vi "Video Settings.vi"(11 "Codec Names":string[](array[string])) -> (0 "Image Width":i32, 1 "Image Height":i32, 2 "Codec Name":string, 3 "AVI fps":u32=5)   [LabVIEW 2013]
panel:
  in  "Image Width":i32
  in  "Image Height":i32
  in  "AVI fps":u32=5
  in  "Codec Index":i32=1
  in  "stop":bool
  # "Enter Video Settings and\nthen Accept."
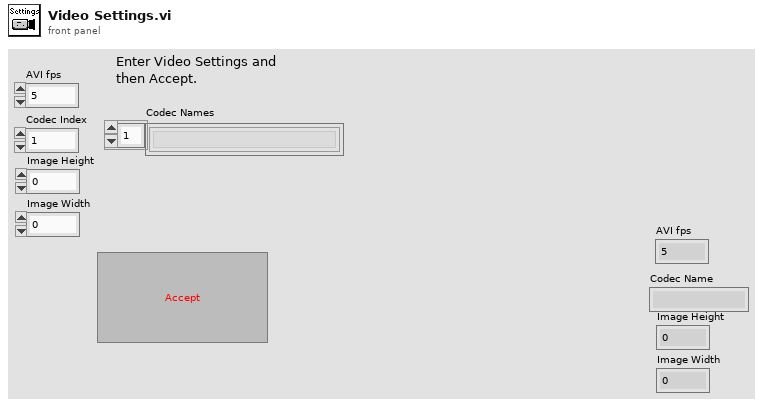
[diagram p1: front panel]
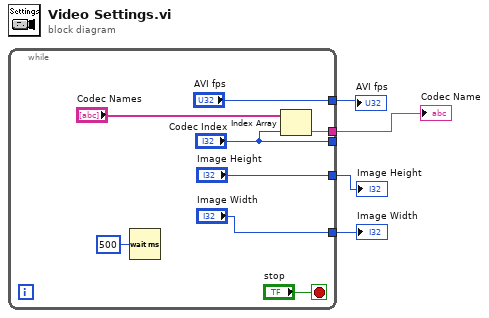
[diagram p0: block diagram]
diagram:
  n1 = while {
    tunnel: ["AVI fps"] -> w4
    tunnel: ["Codec Index"] -> _
    tunnel: ["Image Height"] -> w3
    tunnel: ["Image Width"] -> w2
    tunnel: [w5] -> w1
    stop <- "stop" stop-if-true
    n2 = Wait (ms)(milliseconds to wait=u32 500) -> ()  [unwired: 1 out]
    n3 = Index Array(array="Codec Names", index="Codec Index") -> (element=w5:string)
  }
  "AVI fps" <- w4
  "Image Height" <- w3
  "Image Width" <- w2
  "Codec Name" <- w1
